vi "AppendResult.vi"(7 "head":string[](array[string]), 10 "Configur":T1, 11 "data":string[](array[string])) -> ()   [LabVIEW 2025, in "Test Unit.lvlib"]
uses:
  Test Unit.lvlib
  <vilib>/Test Bench Framework/Test Executive.lvlibp/TestEngine/TestEngine/TestEngine/Typedefs/TestEngine Cofiguration.ctl
  <vilib>/Test Bench Framework/Test Executive.lvlibp/TestEngine/TestEngine/TestEngine/Typedefs/Local Report Configuration.ctl
  <vilib>/Test Bench Framework/Test Executive.lvlibp/TestEngine/TestEngine/TestEngine/Report Format.ctl
  <vilib>/Test Bench Framework/Test Executive.lvlibp/TestEngine/TestEngine/TestEngine/Typedefs/Database Configuration.ctl
  <userlib>/_OpenG.lib/file/file.llb/File Exists - Scalar__ogtk.vi
  <vilib>/Utility/file.llb/Read Delimited Spreadsheet (string).vi
  <vilib>/Utility/file.llb/Write Delimited Spreadsheet (string).vi
  <userlib>/_OpenG.lib/file/file.llb/openg_file.lvlib
  <vilib>/Test Bench Framework/Test Executive.lvlibp/TestEngine/TestEngine/TestEngine/Test Engine.lvclass
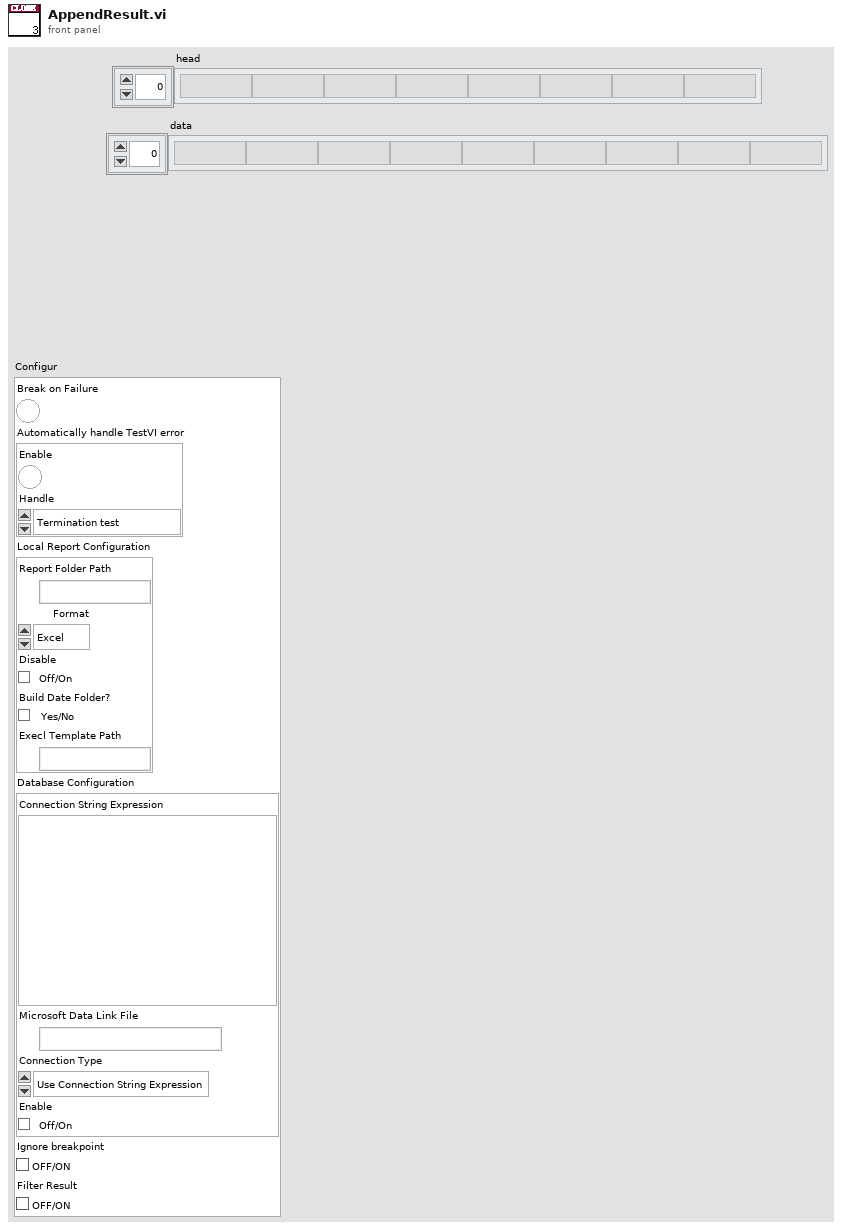
[diagram p1: front panel]
types:
  T1 = typedef "Test Executive.lvlibp/Test Engine.lvlib/Test Engine.lvclass/TestEngine Cofiguration.ctl" = cluster{"Break on Failure":bool, "Automatically handle TestVI error":cluster{"Enable":bool, "Handle":enum16{"Termination test", "Ignore error"}}, "Local Report Configuration":T2, "Database Configuration":T4, "Ignore breakpoint":bool, "Filter Result":bool}
  T2 = typedef "Test Executive.lvlibp/Test Engine.lvlib/Test Engine.lvclass/Local Report Configuration.ctl" = cluster{"Report Folder Path":path, "Format":T3, "Disable":bool, "Build Date Folder?":bool, "Execl Template Path":path}
  T3 = typedef "Test Executive.lvlibp/Test Engine.lvlib/Test Engine.lvclass/Report Format.ctl" = enum16{"Excel", "CSV(Tab)", "CSV(,)", "CSV(;)", "TEXT", "HTML"}
  T4 = typedef "Test Executive.lvlibp/Test Engine.lvlib/Test Engine.lvclass/Database Configuration.ctl" = cluster{"Connection String Expression":string, "Microsoft Data Link File":path, "Connection Type":enum16{"Use Connection String Expression", "Use Microsoft Data Link File"}, "Enable":bool}
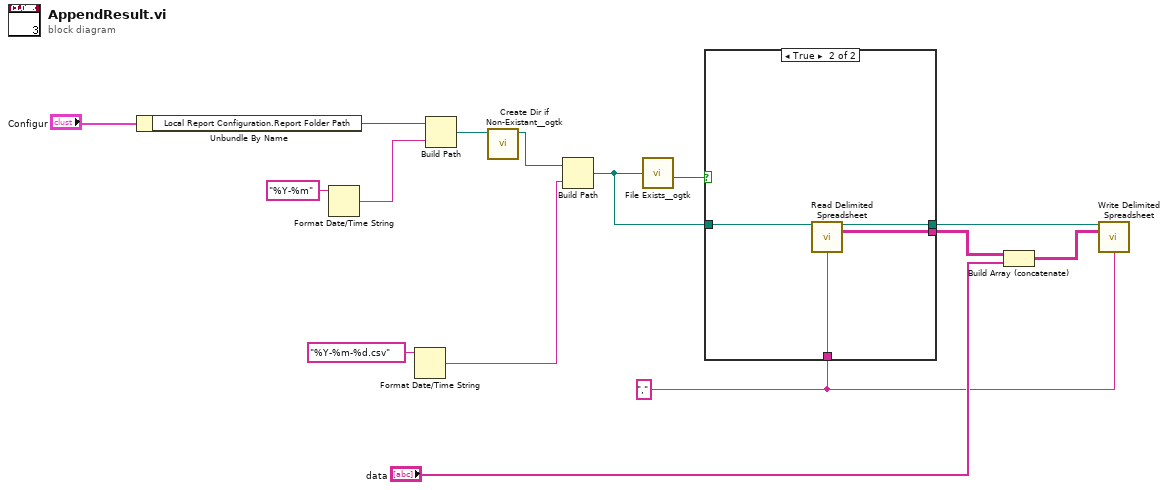
[diagram p0: block diagram]
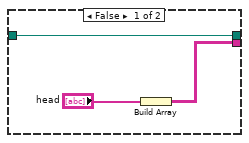
[diagram p2: hidden frame]
diagram:
  w1 = "," ("delimiter (\\t)")
  n1 = Unbundle By Name("Configur") -> ("Local Report Configuration.Report Folder Path"=w13:path)
  n2 = Format Date/Time String(time format string (%c)="%Y-%m") -> (date/time string=w12:string)  [unwired: 2 in]
  n3 = Format Date/Time String(time format string (%c)="%Y-%m-%d.csv") -> (date/time string=w8:string)  [unwired: 2 in]
  n4 = Build Path(base path=w13, name or relative path=w12) -> (appended path=w11:path)
  n5 = call <userlib>:"Create Dir if Non-Existant__ogtk.vi"("Directory Path"=w11) -> ("dup Directory Path"=w9:path)  [unwired: 8 in, 2 out]
  n6 = Build Path(base path=w9, name or relative path=w8) -> (appended path=w6:path)
  n7 = call-poly <userlib>:"File Exists__ogtk.vi"("file path"=w6) -> ("exists"=w7:bool)  [unwired: 6 in, 1 out]
  n8 = case shown="True" w7 {
    tunnel: w6 -> [w17 w22]
    tunnel: [w16 w21] -> w4
    tunnel: [w17 w20] -> w5
    tunnel: w1 -> [_ w19]
    frame False {
      n9 = Build Array("head") -> (w16:string[][])
    }
    frame True {
      n10 = call-poly <vilib>:"Read Delimited Spreadsheet.vi"("file path (dialog if empty)"=w22, "delimiter (\\t)"=w19) -> ("new file path (Not A Path if cancelled)"=w20:path, "all rows"=w21:string[][])  [unwired: 8 in, 4 out]
    }
  }
  n11 = Build Array (concatenate)(w4, "data") -> (w2:string[][])
  n12 = call-poly <vilib>:"Write Delimited Spreadsheet.vi"("file path (dialog if empty)"=w5, "2D data"=w2, "delimiter (\\t)"=w1) -> ()  [unwired: 11 in, 2 out]
